vi "Motor Commands.vi"(8 "error in (no error)":errorcluster, 11 "Command Queue":refnum<queue>) -> (0 "error out":errorcluster)   [LabVIEW 2016]
uses:
  Message Format.ctl
  States.ctl
  <vilib>/addons/zeromq/socket_type.ctl
  <vilib>/addons/zeromq/socket_options.ctl
  <vilib>/addons/zeromq/zmq_context.lvclass
  <vilib>/addons/zeromq/zmq_socket.lvclass
  <vilib>/addons/zeromq/zeromq.lvlib
panel:
  out "data":string
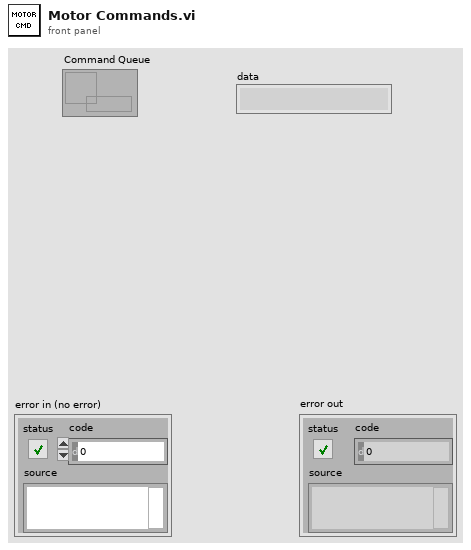
[diagram p1: front panel]
types:
  T1 = typedef "States.ctl" = enum16{"Initialize", "Running", "Exit"}
  T2 = typedef "zeromq.lvlib/socket_options.ctl" = enum8{"NONE", "ZMQ_HWM", "<2>", "ZMQ_SWAP", "ZMQ_AFFINITY", "ZMQ_IDENTITY", "ZMQ_SUBSCRIBE", "ZMQ_UNSUBSCRIBE", "ZMQ_RATE", "ZMQ_RECOVERY_IVL", "ZMQ_MCAST_LOOP", "ZMQ_SNDBUF", "ZMQ_RCVBUF", "ZMQ_RCVMORE", "ZMQ_FD", "ZMQ_EVENTS", "ZMQ_TYPE", "ZMQ_LINGER", "ZMQ_RECONNECT_IVL", "ZMQ_BACKLOG", "ZMQ_RECOVERY_IVL_MSEC", "ZMQ_RECONNECT_IVL_MAX", "ZMQ_MAXMSGSIZE", "ZMQ_SNDHWM", "ZMQ_RCVHWM", "ZMQ_MULTICAST_HOPS", "<26>", "ZMQ_RCVTIMEO", "ZMQ_SNDTIMEO", "<29>", "<30>", "ZMQ_IPV4ONLY", "ZMQ_LAST_ENDPOINT", "ZMQ_ROUTER_MANDATORY", "ZMQ_TCP_KEEPALIVE", "ZMQ_TCP_KEEPALIVE_CNT", "ZMQ_TCP_KEEPALIVE_IDLE", "ZMQ_TCP_KEEPALIVE_INTVL", "ZMQ_TCP_ACCEPT_FILTER", "ZMQ_DELAY_ATTACH_ON_CONNECT", "ZMQ_XPUB_VERBOSE"}
  T3 = typedef "zeromq.lvlib/socket_type.ctl" = enum8{"ZMQ_PAIR", "ZMQ_PUB", "ZMQ_SUB", "ZMQ_REQ", "ZMQ_REP", "ZMQ_DEALER", "ZMQ_ROUTER", "ZMQ_PULL", "ZMQ_PUSH", "ZMQ_XPUB", "ZMQ_XSUB"}
  T4 = typedef "Message Format.ctl" = cluster{"header":string, "data":variant}
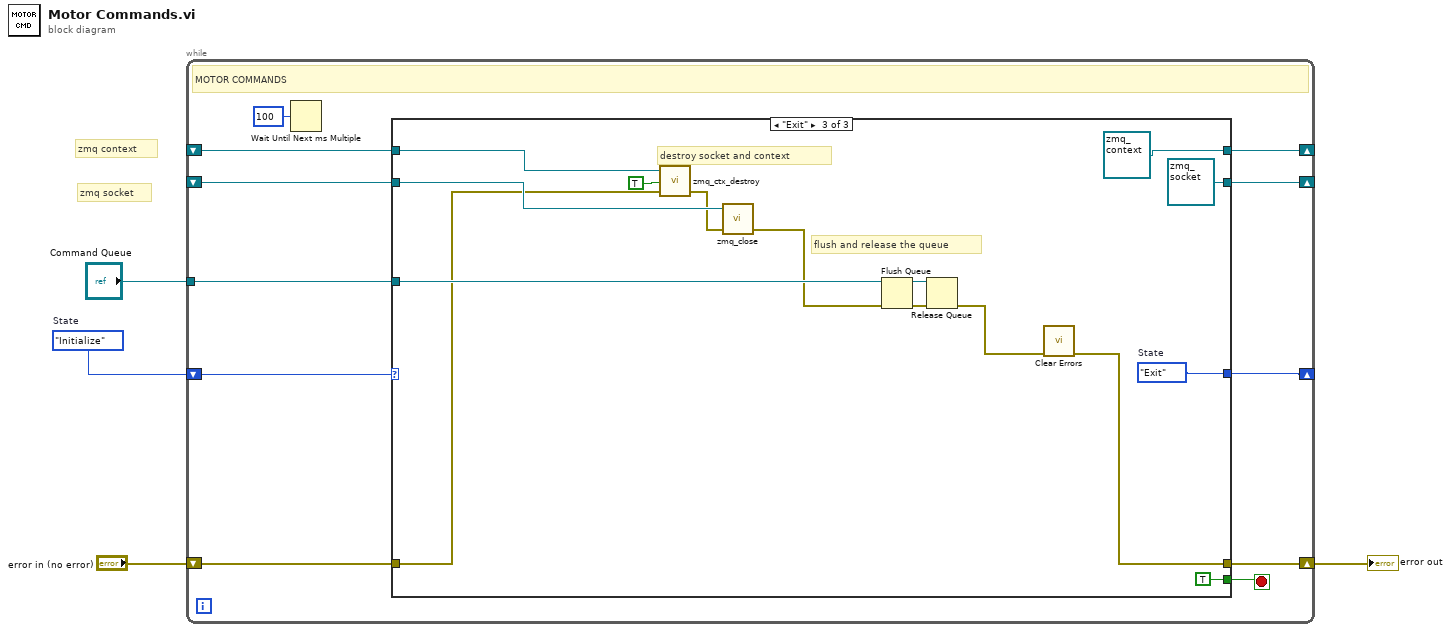
[diagram p0: block diagram]
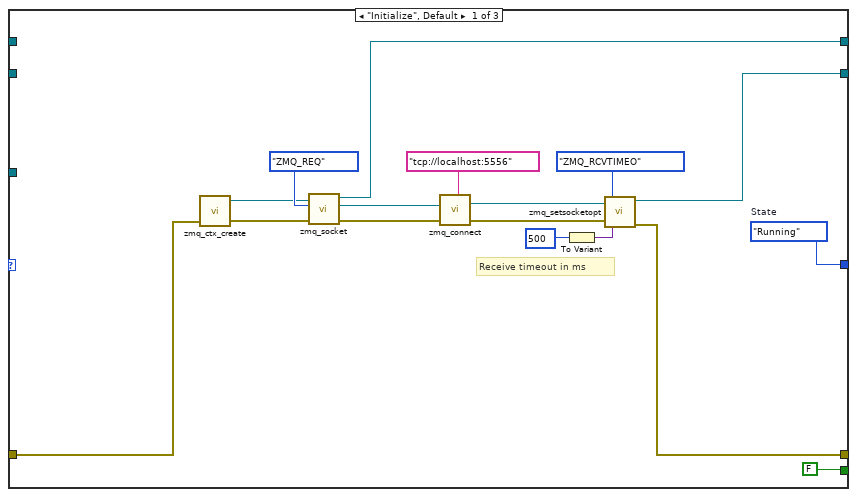
[diagram p2: hidden frame]
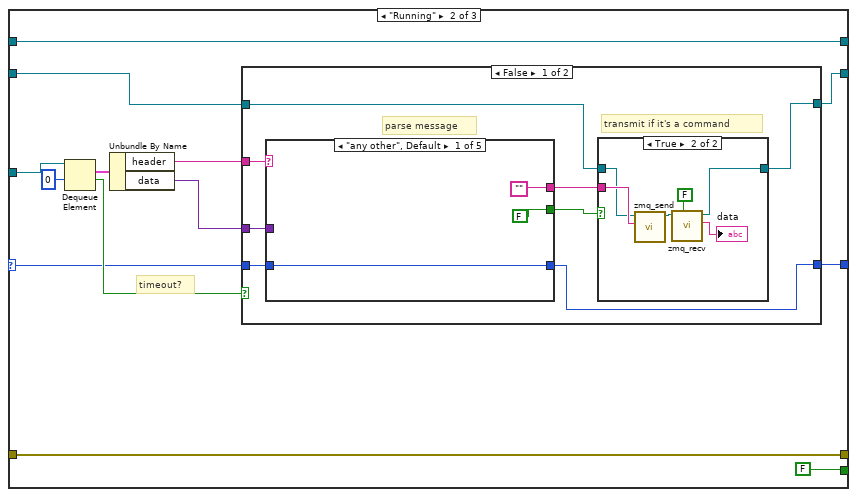
[diagram p3: hidden frame]
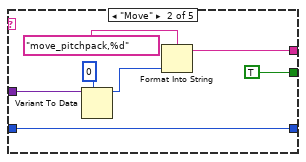
[diagram p5: hidden frame]
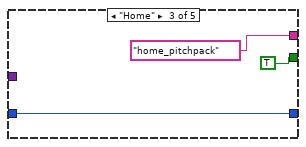
[diagram p6: hidden frame]
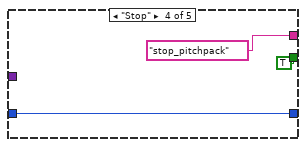
[diagram p7: hidden frame]
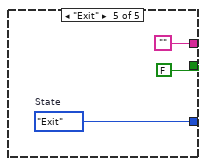
[diagram p8: hidden frame]
diagram:
  w2 = States."Initialize"  # State
  # "zmq socket"
  # "zmq context"
  n1 = while {
    shift-right: [w15] -> w1
    shift-left: "error in (no error)" -> [w8]
    shift-right: [w13] -> _
    shift-left: _ -> [w12]
    shift-right: [w11] -> _
    shift-left: _ -> [w10]
    tunnel: "Command Queue" -> [w6]
    shift-right: [w7] -> _
    shift-left: w2 -> [w9]
    stop <- w5 stop-if-true
    # "MOTOR COMMANDS"
    n2 = Wait Until Next ms Multiple(millisecond multiple=u32 100) -> ()  [unwired: 1 out]
    n3 = case shown="\"Exit\"" w9 {
      selector: w9 -> [_ w37 _]
      tunnel: [w32 w33 w85] -> w15
      tunnel: [w31 w36 refnum<class "zmq_socket.lvclass"> refnum ("socket out")] -> w13
      tunnel: w12 -> [_ w38 w93]
      tunnel: [w20 w45 refnum<class "zmq_context.lvclass"> refnum ("context out")] -> w11
      tunnel: w10 -> [_ w45 w96]
      tunnel: w8 -> [w21 w33 w84]
      tunnel: [w17 w35 w94] -> w7
      tunnel: w6 -> [_ w42 w90]
      tunnel: [FALSE FALSE TRUE] -> w5
      frame "Initialize", Default {
        w17 = States."Running"  # State
        # "Receive timeout in ms"
        n4 = call <vilib>:"zmq_ctx_create.vi"("error in"=w21) -> ("error out"=w25:errorcluster, "context out"=w22:refnum<class "zmq_context.lvclass">)  [unwired: 3 in]
        n5 = call <vilib>:"zmq_socket.vi"("error in"=w25, "socket type"=socket_type."ZMQ_REQ", "context in"=w22) -> ("error out"=w18:errorcluster, "socket out"=w23:refnum<class "zmq_socket.lvclass">, "context out"=w20:refnum<class "zmq_context.lvclass">)  [unwired: 2 in]
        n6 = call <vilib>:"zmq_connect.vi"("error in"=w18, "endpoint"="tcp://localhost:5556", "socket in"=w23) -> ("error out"=w27:errorcluster, "socket out"=w19:refnum<class "zmq_socket.lvclass">)  [unwired: 1 in]
        n7 = To Variant(anything=500) -> (Variant=w30:variant)
        n8 = call <vilib>:"zmq_setsocketopt.vi"("error in"=w27, "value"=w30, "option"=socket_options."ZMQ_RCVTIMEO", "socket in"=w19) -> ("error out"=w32:errorcluster, "socket out"=w31:refnum<class "zmq_socket.lvclass">)  [unwired: 2 in]
      }
      frame "Running" {
        # "timeout?"
        n9 = Dequeue Element(queue=w42, timeout in ms (-1)=0) -> (element=w43:T4, timed out?=w41:bool)  [unwired: 1 in, 2 out]
        n10 = Unbundle By Name(w43) -> ("header"=w40:string, "data"=w39:variant)
        n11 = case shown="False" w41 {
          tunnel: w40 -> [w53 _]
          tunnel: w39 -> [w50 _]
          tunnel: w38 -> [w49 w80]
          tunnel: w37 -> [w48 w81]
          tunnel: [w47 w80] -> w36
          tunnel: [w46 w81] -> w35
          frame False {
            # "parse message"
            # "transmit if it's a command"
            n12 = case shown="\"any other\", Default" w53 {
              tunnel: [FALSE TRUE TRUE TRUE FALSE] -> w52
              tunnel: ["" w68 "home_pitchpack" "stop_pitchpack" ""] -> w51
              tunnel: w50 -> [_ w70 _ _ _]
              tunnel: w48 -> [w61 w66 w71 w74 _]
              tunnel: [w61 w66 w71 w74 w77] -> w46
              frame "any other", Default {
              }
              frame "Move" {
                n13 = Variant To Data(type=0, Variant=w70) -> (data=w64:i32)  [unwired: 1 in, 1 out]
                n14 = Format Into String(format string="move_pitchpack,%d", w64) -> (resulting string=w68:string)  [unwired: 2 in, 1 out]
              }
              frame "Home" {
              }
              frame "Stop" {
              }
              frame "Exit" {
                w77 = States."Exit"  # State
              }
            }
            n15 = case shown="True" w52 {
              tunnel: w51 -> [_ w58]
              tunnel: w49 -> [w54 w56]
              tunnel: [w54 w55] -> w47
              frame False {
              }
              frame True {
                n16 = call <vilib>:"zmq_send.vi"("data"=w58, "socket in"=w56) -> ("socket out"=w60:refnum<class "zmq_socket.lvclass">)  [unwired: 5 in, 1 out]
                n17 = call <vilib>:"zmq_recv.vi"("no block? (F)"=FALSE, "socket in"=w60) -> ("data"=→"data":string, "socket out"=w55:refnum<class "zmq_socket.lvclass">)  [unwired: 3 in, 3 out]
              }
            }
          }
          frame True {
          }
        }
      }
      frame "Exit" {
        w94 = States."Exit"  # State
        # "flush and release the queue"
        # "destroy socket and context"
        n18 = call <vilib>:"zmq_ctx_destroy.vi"("error in"=w84, "reap? (F)"=TRUE, "context in"=w96) -> ("error out"=w87:errorcluster)  [unwired: 2 in]
        n19 = call <vilib>:"zmq_close.vi"("error in"=w87, "socket"=w93) -> ("error out"=w83:errorcluster)  [unwired: 3 in]
        n20 = Flush Queue(queue=w90, error in (no error)=w83) -> (queue out=w88:refnum<queue>, error out=w82:errorcluster)  [unwired: 1 out]
        n21 = Release Queue(queue=w88, error in (no error)=w82) -> (error out=w86:errorcluster)  [unwired: 1 in, 2 out]
        n22 = call <vilib>:"Clear Errors.vi"("error in (no error)"=w86) -> ("error out"=w85:errorcluster)  [unwired: 5 in, 1 out]
      }
    }
  }
  "error out" <- w1
